vi "Set stack data.vi"(8 "error in (no error)":errorcluster, 9 "Common data array":string[](array[string]), 10 "Is module?":bool, 11 "Stack in":refnum<class "Stack.lvclass">) -> (0 "error out":errorcluster, 3 "Stack out":refnum<class "Stack.lvclass">)   [LabVIEW 2022 SP3, in "Stack.lvclass"]
uses:
  Stack.lvclass
  Stack.lvclass/Stack.ctl
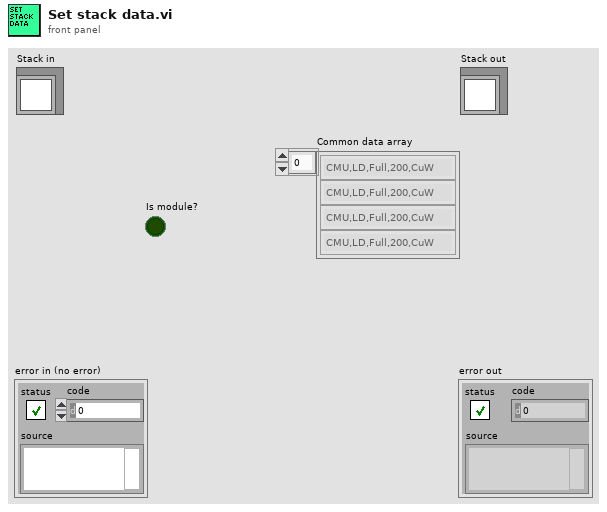
[diagram p1: front panel]
types:
  T1 = cluster{"Common data array[0]":string, "Common data array[1]":string, "Common data array[2]":string, "Common data array[3]":string, "Common data array[4]":string, "Common data array[5]":string, "Common data array[6]":string, "Common data array[7]":string, "Common data array[8]":string}
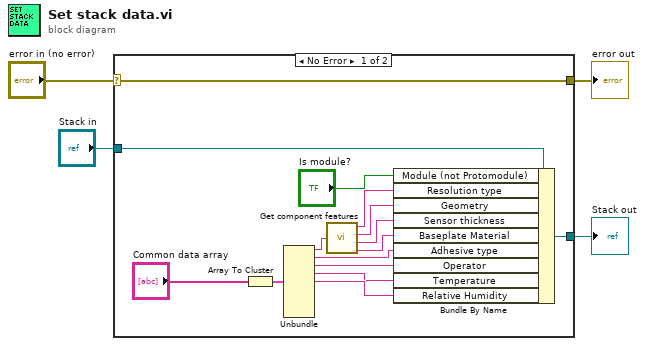
[diagram p0: block diagram]
diagram:
  n1 = case shown="No Error" "error in (no error)" {
    selector: "error in (no error)" -> [w19 w21]
    tunnel: [w19 w21] -> w3
    tunnel: [w18 w20] -> w1
    tunnel: "Stack in" -> [w17 w20]
    frame No Error {
      n2 = Array To Cluster(array="Common data array") -> (cluster=w11:T1)
      n3 = Unbundle(w11) -> ("Common data array[0]"=w10:string, "Common data array[1]"=w9:string, "Common data array[2]"=w8:string, "Common data array[3]"=w6:string, "Common data array[4]"=w7:string)  [unwired: 4 out]
      n4 = call "Get component features.vi"("Module Type"=w10) -> ("Resolution"=w15:string, "Geometry"=w16:string, "Sensor thickness"=w14:string, "BP Type"=w13:string)  [unwired: 1 in, 1 out]
      n5 = Bundle By Name(cluster=w17, "Module (not Protomodule)"="Is module?", "Resolution type"=w15, "Geometry"=w16, "Sensor thickness"=w14, "Baseplate Material"=w13, "Adhesive type"=w9, "Operator"=w8, "Temperature"=w6, "Relative Humidity"=w7) -> (w18:refnum<class "Stack.lvclass">)
    }
    frame Error {
    }
  }
  "error out" <- w3
  "Stack out" <- w1
